vi "ReadByteInUART.vi"(11 "FPGA VI Reference In":refnum<k20>) -> (0 "OverRunError":bool, 1 "Did Read Byte":bool, 2 "Byte Value":u8, 3 "FPGA VI Reference Out":refnum<k20>)   [LabVIEW 2012]
uses:
  <vilib>/Utility/error.llb/Error Cluster From Error Code.vi
  <vilib>/RVI Host/nirviSupport.llb/nirviErrorClusterFromErrorCode.vi
  <vilib>/rvi/errors/niLvFpgaAdjustHostInterfaceError.vi
  <vilib>/rvi/interface/nirviMethod/nirviMethod.xnode
  <vilib>/rvi/interface/nirviReadWriteControl/nirviReadWriteControl.xnode
  NiFpgaLv.dll
  <vilib>/rvi/interface/Simulation/niFpgaSimulationCallBeginRW.vi
  <vilib>/rvi/interface/nirviMethod/StockFPGA_InlinedMethodWaitForSingleIRQ.vi
  <vilib>/FPGAPlugInAG/Dynamic/niLvFpga_WaitOnIrq_Dynamic.vi
  <vilib>/FPGAPlugInAG/Dynamic/niLvFpga_AcknowledgeIrq_Dynamic.vi
panel:
  out "error out":errorcluster
  in  "error in":errorcluster
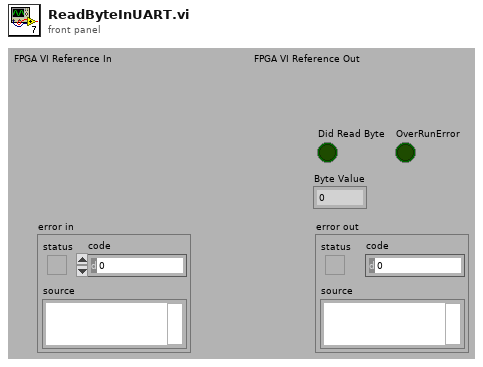
[diagram p1: front panel]
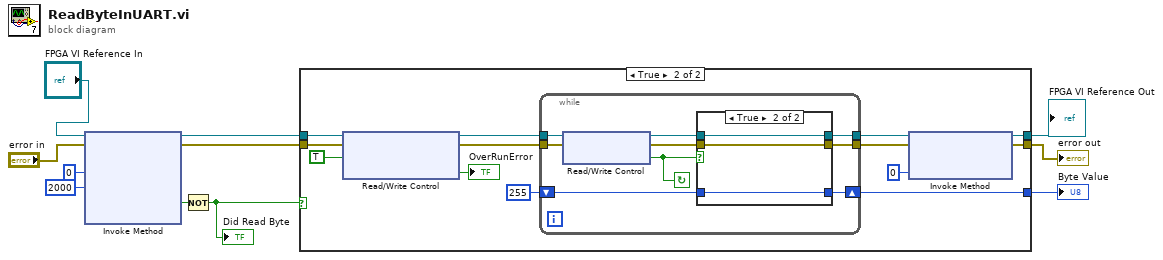
[diagram p0: block diagram]
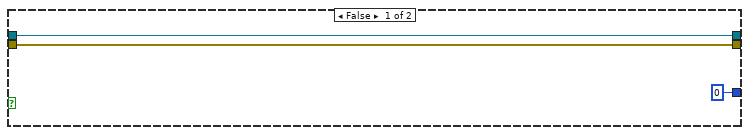
[diagram p2: hidden frame]
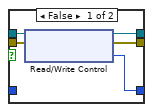
[diagram p3: hidden frame]
diagram:
  n1 = xnode "Invoke Method"("FPGA VI Reference In"="FPGA VI Reference In", "error in"="error in", "IRQ Number(s)"=0, "Timeout (ms)"=2000) -> ("FPGA VI Reference Out"=w6:refnum<k20>, "error out"=w5:errorcluster, "Timed Out"=w4:bool)  [unwired: 1 out]
  n2 = Not(x=w4) -> (.not. x?=w3:bool)
  "Did Read Byte" <- w3
  n3 = case shown="True" w3 {
    tunnel: [u8 0 ("Receive Byte") w27] -> w11
    tunnel: [w13 w16] -> w10
    tunnel: [w12 w17] -> w1
    tunnel: w6 -> [w12 w21]
    tunnel: w5 -> [w13 w20]
    frame False {
    }
    frame True {
      n4 = xnode "Read/Write Control"("FPGA VI Reference In"=w21, "error in"=w20, "UART.Receive"=TRUE ("Read Uart Byte")) -> ("FPGA VI Reference Out"=w25:refnum<k20>, "error out"=w24:errorcluster, "UART.Overrun Error"=→"OverRunError":bool)
      n5 = while {
        tunnel: w25 -> [w36]
        tunnel: w24 -> [w35]
        tunnel: [w32] -> w18
        tunnel: [w31] -> w15
        shift-right: [w30] -> w27
        shift-left: u8 255 ("Receive Byte") -> [w29]
        stop <- w28 continue-if-true
        n6 = xnode "Read/Write Control"("FPGA VI Reference In"=w36, "error in"=w35) -> ("FPGA VI Reference Out"=w34:refnum<k20>, "error out"=w33:errorcluster, "UART.Receive"=w28:bool)
        n7 = case shown="True" w28 {
          tunnel: w34 -> [w41 w43]
          tunnel: w33 -> [w40 w42]
          tunnel: [w39 w43] -> w32
          tunnel: [w38 w42] -> w31
          tunnel: [w37 w44] -> w30
          tunnel: w29 -> [_ w44]
          frame False {
            n8 = xnode "Read/Write Control"("FPGA VI Reference In"=w41, "error in"=w40) -> ("FPGA VI Reference Out"=w39:refnum<k20>, "error out"=w38:errorcluster, "UART.Rx Data"=w37:u8)
          }
          frame True {
          }
        }
      }
      n9 = xnode "Invoke Method"("FPGA VI Reference In"=w18, "error in"=w15, "IRQ Number(s)"=0) -> ("FPGA VI Reference Out"=w17:refnum<k20>, "error out"=w16:errorcluster)
    }
  }
  "Byte Value" <- w11
  "error out" <- w10
  "FPGA VI Reference Out" <- w1
